vi "get_matched_issues.vi"(10 "id":i32, 11 "matched set":set{cluster{"CLZ ID":i32, "CV ID":i32}}(c389)) -> (3 "matched cv ids":i32[](array[numeric]))   [LabVIEW 2024, in "CLZ_to_ComicVine.lvlib"]
uses:
  CLZ_to_ComicVine.lvlib
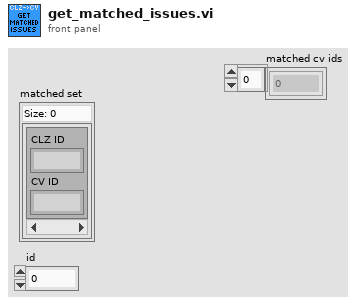
[diagram p1: front panel]
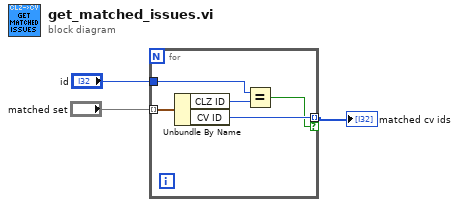
[diagram p0: block diagram]
diagram:
  n1 = for {
    tunnel: "matched set" -> [w8] mode=indexing
    tunnel: "id" -> [w6]
    tunnel: [w5] -> w1 mode=indexing if=w4
    n2 = Unbundle By Name(w8) -> ("CLZ ID"=w7:i32, "CV ID"=w5:i32)
    n3 = Equal?(x=w6, y=w7) -> (x = y?=w4:bool)
  }
  "matched cv ids" <- w1
